vi "Get All Refs.vi"(8 "error in (no error)":errorcluster, 10 "This VI":refnum<vi>, 11 "Control in":refnum<vi>) -> (0 "error out":errorcluster, 1 "Controls[]":refnum<vi>[](array[refnum]), 5 "Label Array":string[](array[string]))   [LabVIEW 2020]
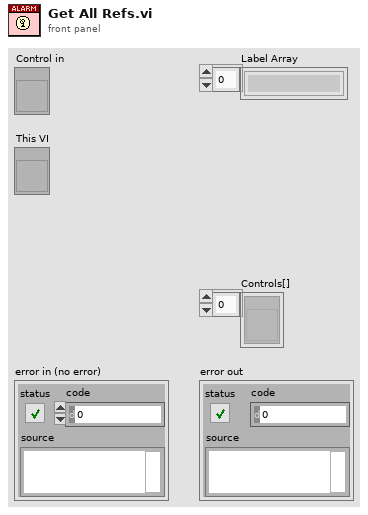
[diagram p1: front panel]
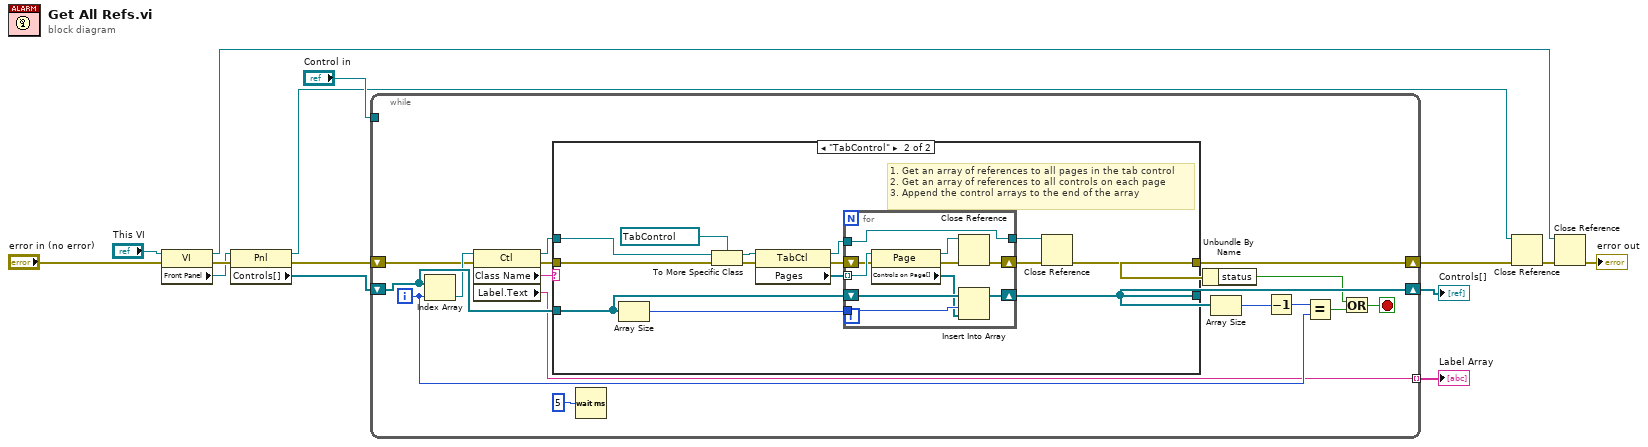
[diagram p0: block diagram]
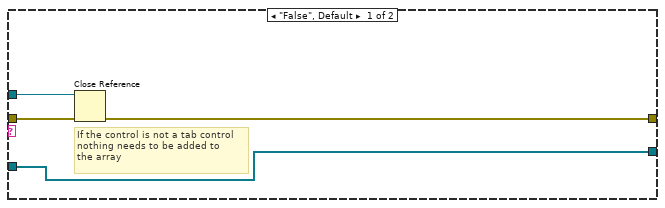
[diagram p2: hidden frame]
diagram:
  n1 = property class="VI"(reference="This VI", error in="error in (no error)") -> (reference out=w1:refnum<vi>, error out=w9:errorcluster, "Front Panel"=w8:refnum<vi>)
  n2 = property class="Pnl"(reference=w8, error in=w9) -> (reference out=w2:refnum<vi>, error out=w10:errorcluster, "Controls[]"=w7:refnum<vi>[])
  n3 = while {
    shift-right: [w22] -> w13
    shift-left: w7 -> [w28]
    tunnel: [w19] -> w6 mode=indexing
    shift-right: [w18] -> w4
    shift-left: w10 -> [w21]
    tunnel: "Control in" -> [_]
    i -> [w23]
    stop <- w16 stop-if-true
    n4 = Index Array(array=w28, index=w23) -> (element=w24:refnum<vi>)
    n5 = property class="Ctl"(reference=w24, error in=w21) -> (reference out=w29:refnum<vi>, error out=w20:errorcluster, "Class Name"=w27:string, "Label.Text"=w19:string)
    n6 = case shown="\"TabControl\"" w27 {
      tunnel: w29 -> [w33 w48]
      tunnel: w28 -> [w34 w44]
      tunnel: [w34 w45] -> w22
      tunnel: w20 -> [w32 w41]
      tunnel: [w31 w37] -> w18
      frame "False", Default {
        # "If the control is not a tab control\nnothing needs to be added to\nthe array"
        n7 = Close Reference(reference=w33, error in (no error)=w32) -> (error out=w31:errorcluster)
      }
      frame "TabControl" {
        # "1. Get an array of references to all pages in the tab control\n2. Get an array of references to all controls on each page\n3. Append the control arrays to the end of the array"
        n8 = Array Size(array=w44) -> (size(s)=w42:i32)
        n9 = To More Specific Class(target class=refnum<vi> refnum ("Tab Control"), reference=w48, error in=w41) -> (specific class reference=w47:refnum<vi>, error out=w40:errorcluster)
        n10 = property class="TabCtl"(reference=w47, error in=w40) -> (reference out=w38:refnum<vi>, error out=w39:errorcluster, "Pages"=w46:refnum<vi>[])
        n11 = for {
          tunnel: w46 -> [w58] mode=indexing
          tunnel: w42 -> [w56]
          shift-right: [w57] -> w45
          shift-left: w44 -> [w55]
          tunnel: w38 -> [w52]
          tunnel: [w52] -> w36
          shift-right: [w49] -> w35
          shift-left: w39 -> [w53]
          n12 = property class="Page"(reference=w58, error in=w53) -> (reference out=w51:refnum<vi>, error out=w50:errorcluster, "Controls on Page[]"=w54:refnum<vi>[])
          n13 = Close Reference(reference=w51, error in (no error)=w50) -> (error out=w49:errorcluster)
          n14 = Insert Into Array(array=w55, index=w56, new element=w54) -> (w57:refnum<vi>[])
        }
        n15 = Close Reference(reference=w36, error in (no error)=w35) -> (error out=w37:errorcluster)
      }
    }
    n16 = Wait (ms)(milliseconds to wait=u32 5) -> ()  [unwired: 1 out]
    n17 = Unbundle By Name(w18) -> ("status"=w15:bool)
    n18 = Array Size(array=w22) -> (size(s)=w26:i32)
    n19 = Decrement(x=w26) -> (x-1=w25:i32)
    n20 = Equal?(x=w25, y=w23) -> (x = y?=w17:bool)
    n21 = Or(x=w15, y=w17) -> (x .or. y?=w16:bool)
  }
  "Controls[]" <- w13
  "Label Array" <- w6
  n22 = Close Reference(reference=w2, error in (no error)=w4) -> (error out=w5:errorcluster)
  n23 = Close Reference(reference=w1, error in (no error)=w5) -> (error out=→"error out":errorcluster)
